vi "LimitsVisible.vi"(8 "error in (no error)":errorcluster, 10 "visible?":bool, 11 "PredictiveMaintenance in":refnum<class "PredictiveMaintenance.lvclass">) -> (0 "error out":errorcluster, 3 "PredictiveMaintenance out":refnum<class "PredictiveMaintenance.lvclass">)   [LabVIEW 2019, in "PredictiveMaintenance.lvlib" / "PredictiveMaintenance.lvclass"]
uses:
  PredictiveMaintenance.lvclass
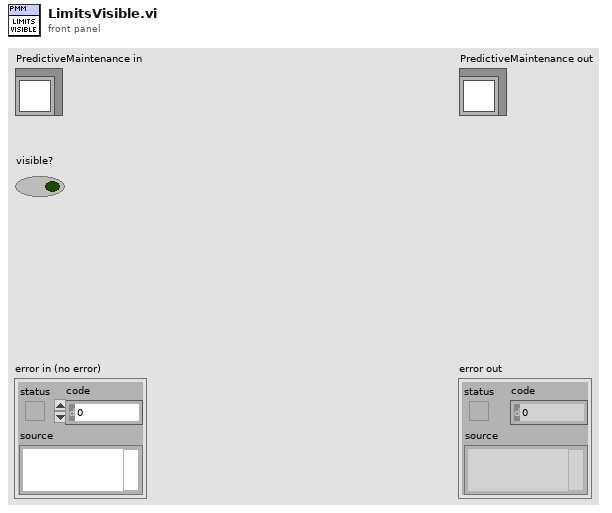
[diagram p1: front panel]
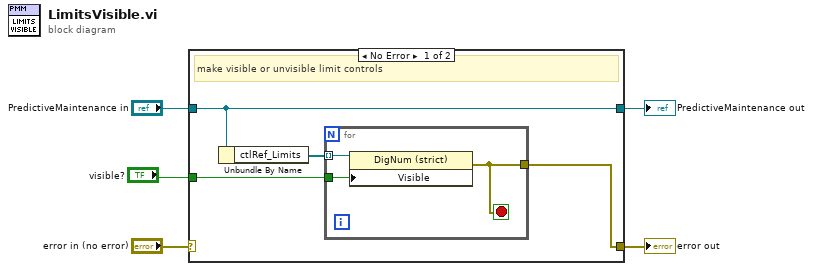
[diagram p0: block diagram]
diagram:
  n1 = case shown="No Error" "error in (no error)" {
    selector: "error in (no error)" -> [_ w14]
    tunnel: [w6 w14] -> w4
    tunnel: [w9 w13] -> w2
    tunnel: "PredictiveMaintenance in" -> [w9 w13]
    tunnel: "visible?" -> [w7 _]
    frame No Error {
      # "make visible or unvisible limit controls"
      n2 = Unbundle By Name(w9) -> ("ctlRef_Limits"=w8:refnum<vi>[])
      n3 = for {
        tunnel: w8 -> [w12] mode=indexing
        tunnel: w7 -> [w11]
        tunnel: [w10] -> w6
        stop <- w10 stop-if-true
        n4 = property class="DigNum (strict)"(reference=w12, "Visible"=w11) -> (error out=w10:errorcluster)  [unwired: 1 in, 1 out]
      }
    }
    frame Error {
    }
  }
  "error out" <- w4
  "PredictiveMaintenance out" <- w2
